vi "EOL CAN_Send_Single_Message_3.vi"(4 "Retries":i32=5, 6 "Msg Wait Time":u32=100, 8 "Rx Arbitration Id":u32=1287 format="%04x", 9 "Tx Arbitration Id":u32=1592 format="%04x", 10 "Tx Msg":u8[](array[numeric])=[2, 26, 156, 255, 255, 255, 255, 255] format="%02x", 11 "NetworkObjHandle":T1) -> (1 "Rx Message":u8[](array[numeric]) format="%02x", 2 "spreadsheet string":string, 3 "Response Good?":bool, 5 "TxRx Data":string[][](array[string]))   [LabVIEW 2018]
uses:
  <vilib>/nican/nican.llb/xobjhandle.ctl
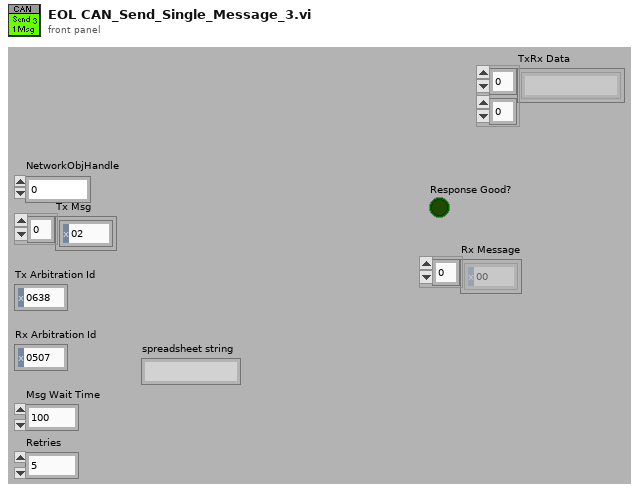
[diagram p1: front panel]
types:
  T1 = typedef "xobjhandle.ctl" = u32
  T2 = cluster{"NetworkObjHandle":T1, "Retry Counter":i32, "Rx Msg":u8[], "Rx Arbitration Id":u32, "Tx Msg":u8[], "Response Good?":bool, "TxRx Data":string[][], "Message Start Timer":u32}
  T3 = typedef "CanFrameTimed.ctl" = cluster{"Timestamp":dbl, "ArbitrationId":u32, "IsRemote":u8, "DataLength":u8, "Data":u8[]}
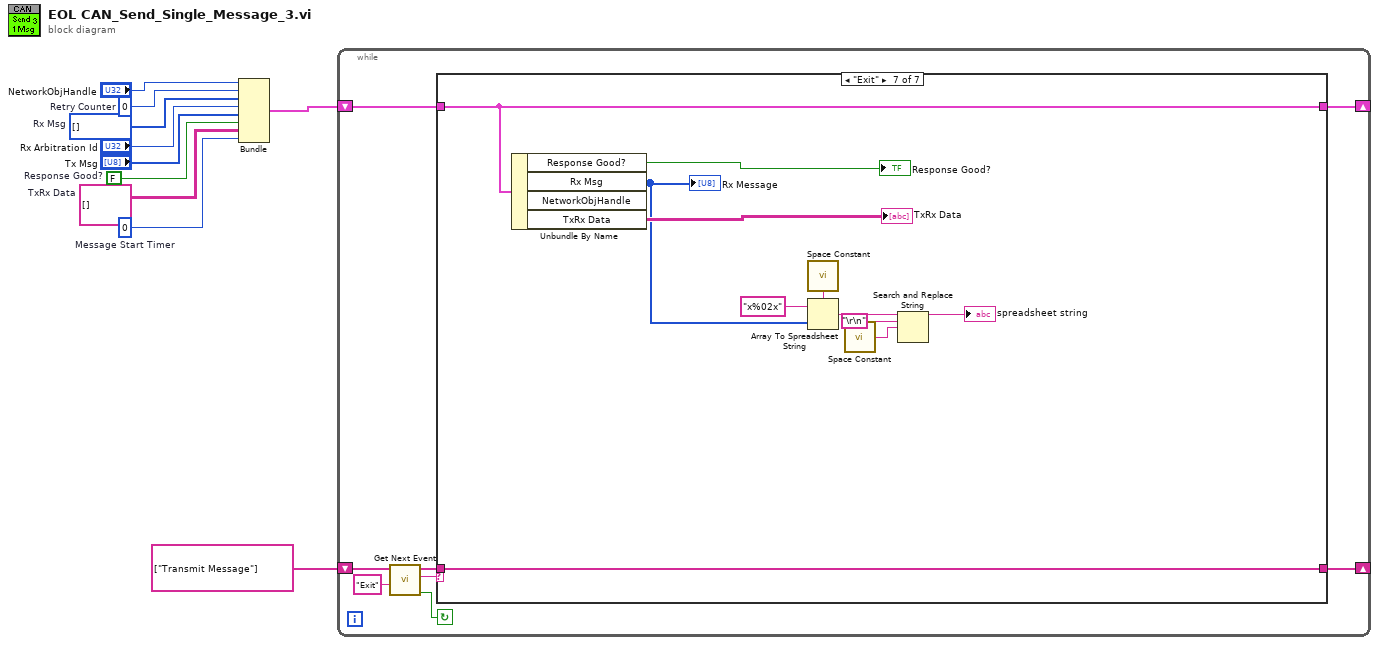
[diagram p0: block diagram]
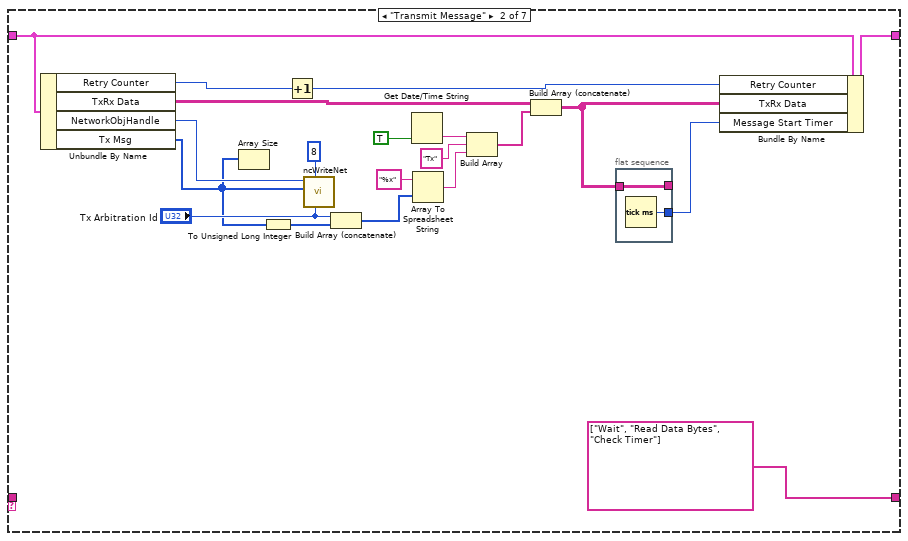
[diagram p3: hidden frame]
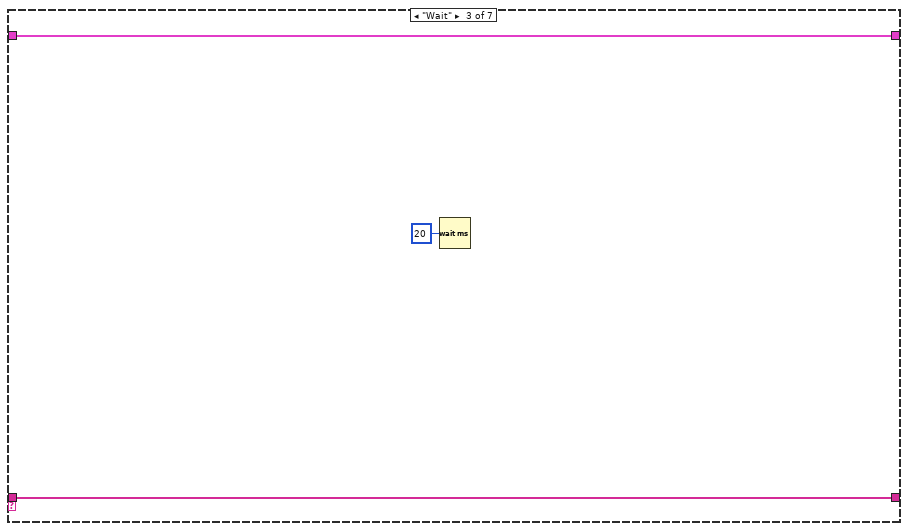
[diagram p4: hidden frame]
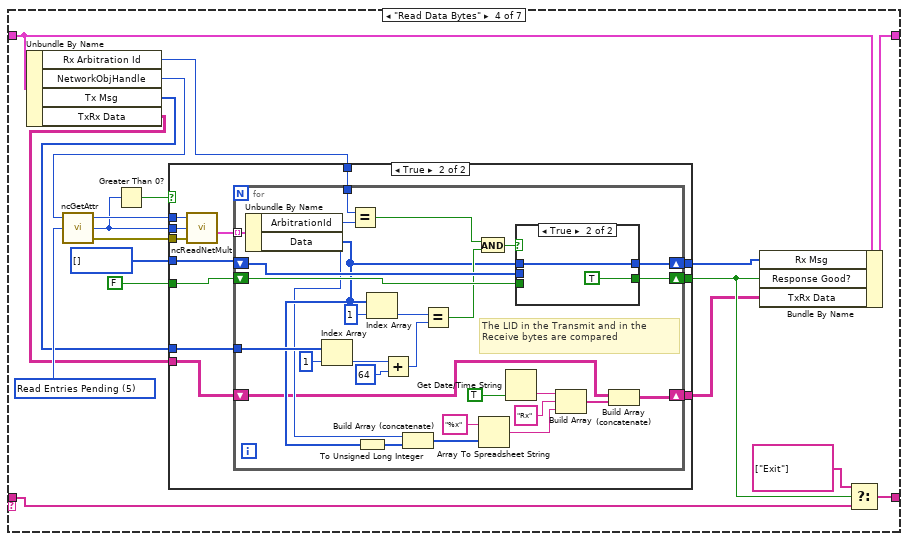
[diagram p5: hidden frame]
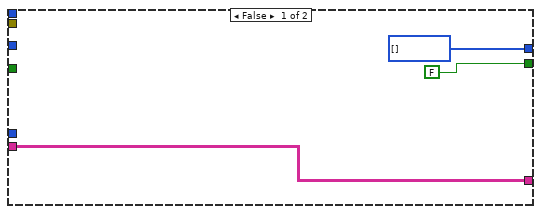
[diagram p6: hidden frame]
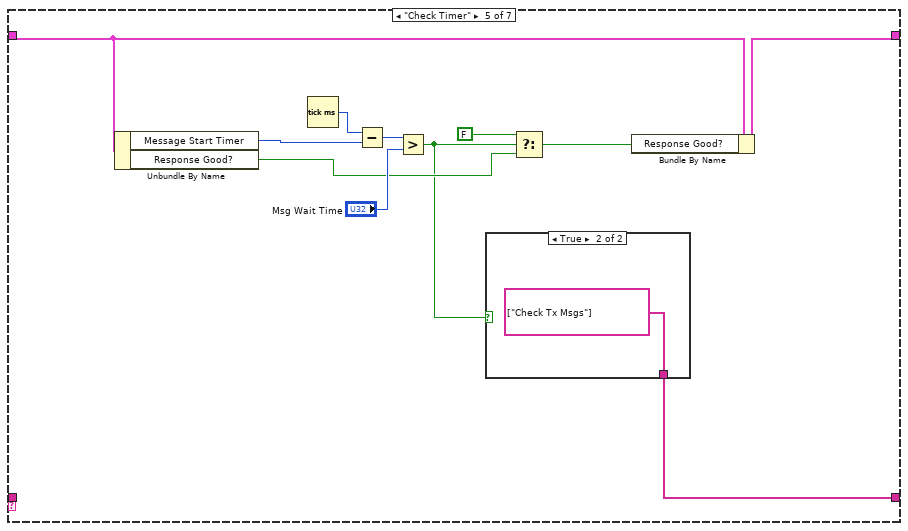
[diagram p8: hidden frame]
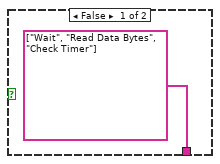
[diagram p9: hidden frame]
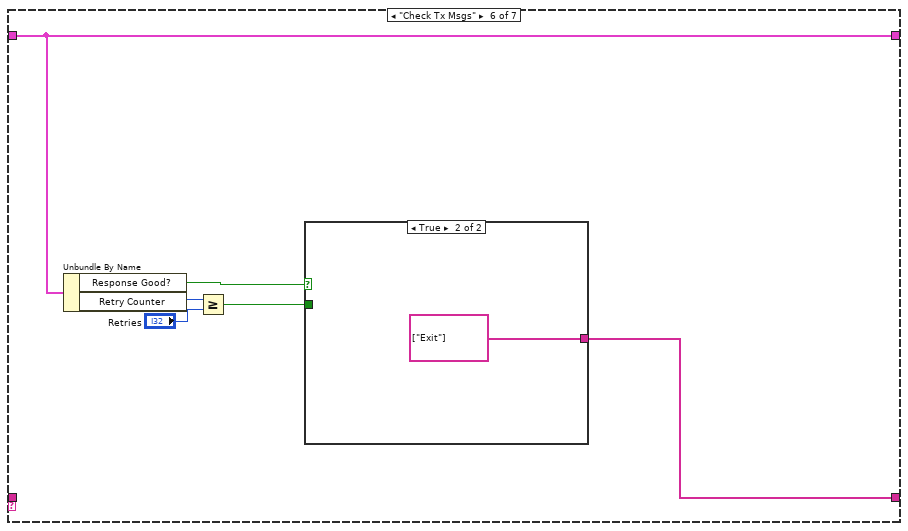
[diagram p10: hidden frame]
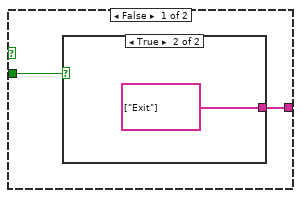
[diagram p11: hidden frame]
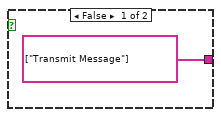
[diagram p12: hidden frame]
diagram:
  w1 = u32 0  # Message Start Timer
  w4 = string[][] []  # TxRx Data
  w6 = FALSE  # Response Good?
  w7 = u8[] []  # Rx Msg
  w9 = 0  # Retry Counter
  n1 = Bundle("NetworkObjHandle"="NetworkObjHandle", "Retry Counter"=w9, "Rx Msg"=w7, "Rx Arbitration Id"="Rx Arbitration Id", "Tx Msg"="Tx Msg", "Response Good?"=w6, "TxRx Data"=w4, "Message Start Timer"=w1) -> (w8:T2)  [unwired: 1 in]
  n2 = while {
    shift-right: [w15] -> _
    shift-left: string[] ["Transmit Message"] ("event queue out") -> [w14]
    shift-right: [w12] -> _
    shift-left: w8 -> [w13]
    stop <- w18 continue-if-true
    n3 = call <userlib>:"Get Next Event.vi"("Exit Event"="Exit", "event queue in"=w14) -> ("Condition (Exit:F)"=w18:bool, "next event"=w17:string, "event queue out"=w16:string[])  [unwired: 3 in]
    n4 = case shown="\"Exit\"" w17 {
      tunnel: w16 -> [w20 _ w43 w51 _ _ w146]
      tunnel: [w20 string[] ["Wait", "Read Data Bytes", "Check Timer"] ("event queue out") w43 w50 w112 w127 w146] -> w15
      tunnel: w13 -> [w19 w38 w44 w59 w114 w125 w145]
      tunnel: [w19 w36 w44 w58 w113 w125 w145] -> w12
      frame "Error", Default {
      }
      frame "Transmit Message" {
        n5 = Unbundle By Name(w38) -> ("Retry Counter"=w39:i32, "TxRx Data"=w22:string[][], "NetworkObjHandle"=w35:T1, "Tx Msg"=w31:u8[])
        n6 = Array Size(array=w31) -> ()  [unwired: 1 out]
        n7 = To Unsigned Long Integer(number=w31) -> (unsigned 32bit integer=w32:u32[])
        n8 = Increment(x=w39) -> (x+1=w37:i32)
        n9 = call <vilib>:"ncWriteNet.vi"("ArbitrationId"="Tx Arbitration Id", "DataLength"=u32 8, "Data"=w31, "ObjHandle in"=w35) -> ()  [unwired: 2 in, 2 out]
        n10 = Build Array (concatenate)("Tx Arbitration Id", w32) -> (w24:u32[])
        n11 = Get Date/Time String(want seconds? (F)=TRUE) -> (time string=w27:string)  [unwired: 2 in, 1 out]
        n12 = Array To Spreadsheet String(array=w24, 3:"%x" ("format string")) -> (spreadsheet string=w29:string)  [unwired: 1 in]
        n13 = Build Array(w27, "Tx" ("format string"), w29) -> (w30:string[])
        n14 = Build Array (concatenate)(w22, w30) -> (w25:string[][])
        n15 = flat-sequence {
          tunnel: w25 -> [w42]
          tunnel: [w42] -> _
          tunnel: [w41] -> w33
          frame #0 {
            n16 = Tick Count (ms)() -> (millisecond timer value=w41:u32)
          }
        }
        n17 = Bundle By Name(cluster=w38, "Retry Counter"=w37, "TxRx Data"=w25, "Message Start Timer"=w33) -> (w36:T2)
      }
      frame "Wait" {
        n18 = Wait (ms)(milliseconds to wait=u32 20) -> ()  [unwired: 1 out]
      }
      frame "Read Data Bytes" {
        w62 = u32 5 items=["(reserved)", "Protocol Version", "Software Version", "Object State", "(reserved)", "Read Entries Pending", "Write Entries Pending", "ReadMult Size for Notification", "Listen Only?", "Self Reception?", "Transmit Error Counter", "Receive Error Counter", "Single Shot Transmit?", "Series 2 Filter Mode", "Series 2 Mask", "Series 2 Comparator", "Serial Number", "Form Factor", "Series", "Transceiver Type", "Interface Number", "Series 2 Error/Arb Capture", "Transceiver Mode", "Transceiver External Outputs", "Transceiver External Inputs", "Start Trigger Behavior", "Log Comm Warnings", "User RTSI Frame", "Transmit Mode", "Log Start Trigger?", "Timestamp Format", "Master Timebase Rate", "Virtual Bus Timing"] ("AttrId")
        n19 = Unbundle By Name(w59) -> ("Rx Arbitration Id"=w48:u32, "NetworkObjHandle"=w54:T1, "Tx Msg"=w53:u8[], "TxRx Data"=w47:string[][])
        n20 = call <vilib>:"ncGetAttr.vi"("AttrId"=w62, "ObjHandle in"=w54) -> ("Error out"=w64:errorcluster, "AttrValue"=w60:u32, "ObjHandle out"=w63:T1)  [unwired: 1 in]
        n21 = Greater Than 0?(x=w60) -> (x > 0?=w61:bool)
        n22 = case shown="True" w61 {
          tunnel: w60 -> [_ w79]
          tunnel: w64 -> [_ w78]
          tunnel: w63 -> [_ w77]
          tunnel: [FALSE w73] -> w52
          tunnel: [u8[] [] ("Data Array") w76] -> w57
          tunnel: u8[] [] ("Data Array") -> [_ w74]
          tunnel: FALSE -> [_ w75]
          tunnel: w53 -> [_ w72]
          tunnel: w48 -> [_ w71]
          tunnel: w47 -> [w65 w69]
          tunnel: [w65 w68] -> w46
          frame False {
          }
          frame True {
            n23 = call <vilib>:"ncReadNetMult.vi"("ObjHandle in"=w77, "Requested Number of Frames"=w79, "Error in"=w78) -> ("Data"=w70:T3[])  [unwired: 3 out]
            n24 = for {
              tunnel: w70 -> [w107] mode=indexing
              shift-right: [w106] -> w76
              shift-left: w74 -> [w105]
              shift-right: [w104] -> w73
              shift-left: w75 -> [w103]
              tunnel: w72 -> [w97]
              tunnel: w71 -> [w93]
              shift-right: [w81] -> w68
              shift-left: w69 -> [w82]
              # "The LID in the Transmit and in the\nReceive bytes are compared"
              n25 = Unbundle By Name(w107) -> ("ArbitrationId"=w89:u32, "Data"=w90:u8[])
              n26 = Index Array(array=w97, index=1) -> (element=w99:u8)
              n27 = Equal?(x=w93, y=w89) -> (x = y?=w101:bool)
              n28 = To Unsigned Long Integer(number=w90) -> (unsigned 32bit integer=w91:u32[])
              n29 = Index Array(array=w90, index=1) -> (element=w96:u8)
              n30 = Add(x=w99, y=u8 64 ("Numeric")) -> (x+y=w95:u8)
              n31 = Build Array (concatenate)(w89, w91) -> (w80:u32[])
              n32 = Equal?(x=w96, y=w95) -> (x = y?=w94:bool)
              n33 = And(x=w101, y=w94) -> (x .and. y?=w102:bool)
              n34 = Array To Spreadsheet String(array=w80, 3:"%x" ("format string")) -> (spreadsheet string=w84:string)  [unwired: 1 in]
              n35 = Get Date/Time String(want seconds? (F)=TRUE) -> (time string=w86:string)  [unwired: 2 in, 1 out]
              n36 = case shown="True" w102 {
                tunnel: w90 -> [_ w110]
                tunnel: [w109 w110] -> w106
                tunnel: w105 -> [w109 _]
                tunnel: [w108 TRUE] -> w104
                tunnel: w103 -> [w108 _]
                frame False {
                }
                frame True {
                }
              }
              n37 = Build Array(w86, "Rx" ("format string"), w84) -> (w83:string[])
              n38 = Build Array (concatenate)(w82, w83) -> (w81:string[][])
            }
          }
        }
        n39 = Bundle By Name(cluster=w59, "Rx Msg"=w57, "Response Good?"=w52, "TxRx Data"=w46) -> (w58:T2)
        n40 = Select(t=string[] ["Exit"], s=w52, f=w51) -> (s? t:f=w50:string[])
      }
      frame "Check Timer" {
        n41 = Unbundle By Name(w114) -> ("Message Start Timer"=w121:u32, "Response Good?"=w117:bool)
        n42 = Tick Count (ms)() -> (millisecond timer value=w122:u32)
        n43 = Subtract(x=w122, y=w121) -> (x-y=w120:u32)
        n44 = Greater?(x=w120, y="Msg Wait Time") -> (0:w115:bool)
        n45 = case shown="True" w115 {
          tunnel: [string[] ["Wait", "Read Data Bytes", "Check Timer"] ("event queue out") string[] ["Check Tx Msgs"] ("Events to Insert")] -> w112
          frame False {
          }
          frame True {
          }
        }
        n46 = Select(t=FALSE, s=w115, f=w117) -> (s? t:f=w116:bool)
        n47 = Bundle By Name(cluster=w114, "Response Good?"=w116) -> (w113:T2)
      }
      frame "Check Tx Msgs" {
        n48 = Unbundle By Name(w125) -> ("Response Good?"=w128:bool, "Retry Counter"=w129:i32)
        n49 = Greater Or Equal?(x=w129, y="Retries") -> (x >= y?=w126:bool)
        n50 = case shown="True" w128 {
          tunnel: [w131 string[] ["Exit"] ("event queue out")] -> w127
          tunnel: w126 -> [w132 _]
          frame False {
            n51 = case shown="True" w132 {
              tunnel: [string[] ["Transmit Message"] ("f") string[] ["Exit"] ("event queue out")] -> w131
              frame False {
              }
              frame True {
              }
            }
          }
          frame True {
          }
        }
      }
      frame "Exit" {
        n52 = Unbundle By Name(w145) -> ("Response Good?"=→"Response Good?":bool, "Rx Msg"=w137:u8[], "TxRx Data"=→"TxRx Data":string[][])  [unwired: 1 out]
        "Rx Message" <- w137
        n53 = call <vilib>:"Space Constant.vi"() -> ("String"=w139:string)
        n54 = Array To Spreadsheet String(delimiter (Tab)=w139, array=w137, 3:"x%02x" ("format string")) -> (spreadsheet string=w138:string)
        n55 = call <vilib>:"Space Constant.vi"() -> ("String"=w141:string)
        n56 = Search and Replace String(input string=w138, search string="\r\n", replace string=w141) -> (result string=→"spreadsheet string":string)  [unwired: 5 in, 3 out]
      }
    }
  }
